vi "4 PulseMeasurements.vi"(2 "4 Pulse Meas Chs":T1={"DI0"="Connector0/DIO0", "DI1"="Connector0/DIO1", "DI2"="Connector0/DIO2", "DI3"="Connector0/DIO3"}, 4 "PulseMeas Timeouts":u32[](array[numeric])=[0, 0, 0, 0]) -> (7 "PulseMeas Packets":u64[](array[numeric]))   [LabVIEW 2010]
uses:
  <vilib>/eio/EIONode/EIONode.xnode
  <vilib>/rvi/eio/nirviEIOImplementation/nirviEIOImplementation.xnode
  <vilib>/rvi/eio/common/nirviEmuClasses.ctl
  <vilib>/rvi/eio/common/nirviEmuTemplateMethod_noerrors.vi
  <vilib>/NI Veristand/FPGA/NI_VS FPGA Support.lvlib
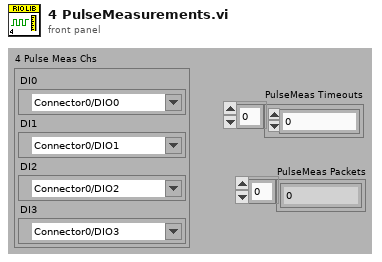
[diagram p1: front panel]
types:
  T1 = cluster{"DI0":refnum<k21>, "DI1":refnum<k21>, "DI2":refnum<k21>, "DI3":refnum<k21>}
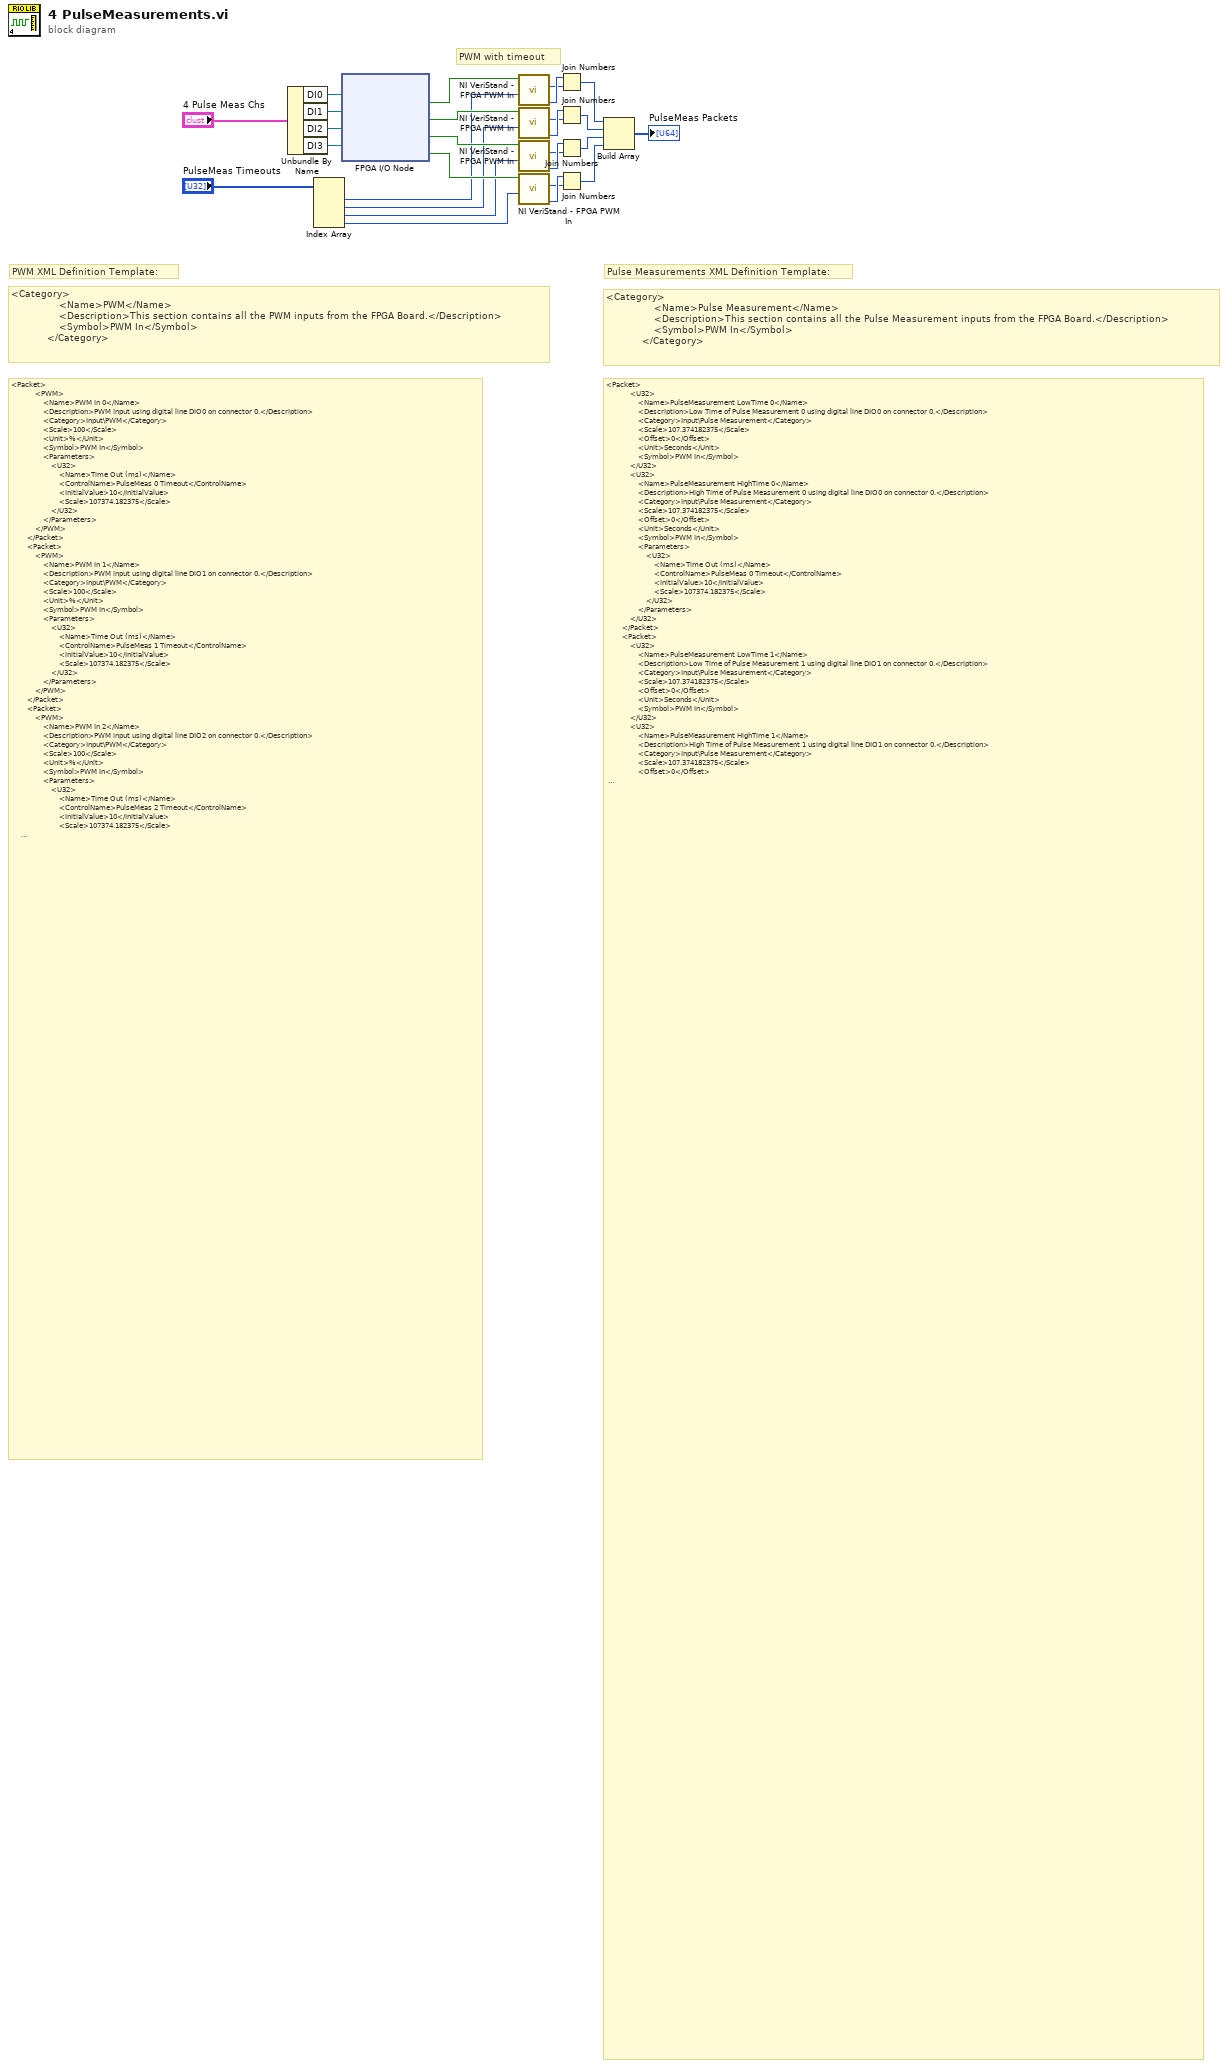
[diagram p0: block diagram]
diagram:
  # "<Category>\n                <Name>PWM</Name>\n                <Description>This section contains all the PWM inputs from the FPGA Board.</Description>\n                <Symbol>PWM In</Symbol>\n            </Category>"
  # "<Category>\n                <Name>Pulse Measurement</Name>\n                <Description>This section contains all the Pulse Measurement inputs from the FPGA Board.</Description>\n                <Symbol>PWM In</Symbol>\n            </Category>"
  # "Pulse Measurements XML Definition Template:"
  # "PWM XML Definition Template:"
  # "<Packet>\n            <PWM>\n                <Name>PWM In 0</Name>\n                <Description>PWM input using digital line DIO0 on connector 0.</Description>\n                <Category>Input\\PWM</Category>\n                <Scale>100</Scale>\n                <Unit>%</Unit>\n                <Symbol>PWM In</Symbol>\n                <Parameters>\n                    <U32>\n                        <Name>Time Out (ms)</Name>\n                        <ControlName>PulseMeas 0 Timeout</ControlName>\n                        <InitialValue>10</InitialValue>\n                        <Scale>107374.182375</Scale>\n                    </U32>\n                </Parameters>\n            </PWM>\n        </Packet>\n        <Packet>\n            <PWM>\n                <Name>PWM In 1</Name>\n                <Description>PWM input using digital line DIO1 on connector 0.</Description>\n                <Category>Input\\PWM</Category>\n                <Scale>100</Scale>\n                <Unit>%</Unit>\n                <Symbol>PWM In</Symbol>\n                <Parameters>\n                    <U32>\n                        <Name>Time Out (ms)</Name>\n                        <ControlName>PulseMeas 1 Timeout</ControlName>\n                        <InitialValue>10</InitialValue>\n                        <Scale>107374.182375</Scale>\n                    </U32>\n                </Parameters>\n            </PWM>\n        </Packet>\n        <Packet>\n            <PWM>\n                <Name>PWM In 2</Name>\n                <Description>PWM input using digital line DIO2 on connector 0.</Description>\n                <Category>Input\\PWM</Category>\n                <Scale>100</Scale>\n                <Unit>%</Unit>\n                <Symbol>PWM In</Symbol>\n                <Parameters>\n                    <U32>\n                        <Name>Time Out (ms)</Name>\n                        <ControlName>PulseMeas 2 Timeout</ControlName>\n                        <InitialValue>10</InitialValue>\n                        <Scale>107374.182375</Scale>\n                    </U32>\n                </Parameters>\n            </PWM>\n        </Packet>\n        <Packet>\n            <PWM>\n                <Name>PWM In 3</Name>\n                <Description>PWM input using digital line DIO3 on connector 0.</Description>\n                <Category>Input\\PWM</Category>\n                <Scale>100</Scale>\n                <Unit>%</Unit>\n                <Symbol>PWM In</Symbol>\n                <Parameters>\n                    <U32>\n                        <Name>Time Out (ms)</Name>\n                        <ControlName>PulseMeas 3 Timeout</ControlName>\n                        <InitialValue>10</InitialValue>\n                        <Scale>107374.182375</Scale>\n                    </U32>\n                </Parameters>\n            </PWM>\n        </Packet>"
  # "<Packet>\n            <U32>\n                <Name>PulseMeasurement LowTime 0</Name>\n                <Description>Low Time of Pulse Measurement 0 using digital line DIO0 on connector 0.</Description>\n                <Category>Input\\Pulse Measurement</Category>\n                <Scale>107.374182375</Scale>\n                <Offset>0</Offset>\n                <Unit>Seconds</Unit>\n                <Symbol>PWM In</Symbol>\n            </U32>\n            <U32>\n                <Name>PulseMeasurement HighTime 0</Name>\n                <Description>High Time of Pulse Measurement 0 using digital line DIO0 on connector 0.</Description>\n                <Category>Input\\Pulse Measurement</Category>\n                <Scale>107.374182375</Scale>\n                <Offset>0</Offset>\n                <Unit>Seconds</Unit>\n                <Symbol>PWM In</Symbol>\n                <Parameters>\n                    <U32>\n                        <Name>Time Out (ms)</Name>\n                        <ControlName>PulseMeas 0 Timeout</ControlName>\n                        <InitialValue>10</InitialValue>\n                        <Scale>107374.182375</Scale>\n                    </U32>\n                </Parameters>\n            </U32>\n        </Packet>\n        <Packet>\n            <U32>\n                <Name>PulseMeasurement LowTime 1</Name>\n                <Description>Low Time of Pulse Measurement 1 using digital line DIO1 on connector 0.</Description>\n                <Category>Input\\Pulse Measurement</Category>\n                <Scale>107.374182375</Scale>\n                <Offset>0</Offset>\n                <Unit>Seconds</Unit>\n                <Symbol>PWM In</Symbol>\n            </U32>\n            <U32>\n                <Name>PulseMeasurement HighTime 1</Name>\n                <Description>High Time of Pulse Measurement 1 using digital line DIO1 on connector 0.</Description>\n                <Category>Input\\Pulse Measurement</Category>\n                <Scale>107.374182375</Scale>\n                <Offset>0</Offset>\n                <Unit>Seconds</Unit>\n                <Symbol>PWM In</Symbol>\n                <Parameters>\n                    <U32>\n                        <Name>Time Out (ms)</Name>\n                        <ControlName>PulseMeas 1 Timeout</ControlName>\n                        <InitialValue>10</InitialValue>\n                        <Scale>107374.182375</Scale>\n                    </U32>\n                </Parameters>\n            </U32>\n        </Packet>\n        <Packet>\n            <U32>\n                <Name>PulseMeasurement LowTime 2</Name>\n                <Description>Low Time of Pulse Measurement 2 using digital line DIO2 on connector 0.</Description>\n                <Category>Input\\Pulse Measurement</Category>\n                <Scale>107.374182375</Scale>\n                <Offset>0</Offset>\n                <Unit>Seconds</Unit>\n                <Symbol>PWM In</Symbol>\n            </U32>\n            <U32>\n                <Name>PulseMeasurement HighTime 2</Name>\n                <Description>High Time of Pulse Measurement 2 using digital line DIO2 on connector 0.</Description>\n                <Category>Input\\Pulse Measurement</Category>\n                <Scale>107.374182375</Scale>\n                <Offset>0</Offset>\n                <Unit>Seconds</Unit>\n                <Symbol>PWM In</Symbol>\n                <Parameters>\n                    <U32>\n                        <Name>Time Out (ms)</Name>\n                        <ControlName>PulseMeas 2 Timeout</ControlName>\n                        <InitialValue>10</InitialValue>\n                        <Scale>107374.182375</Scale>\n                    </U32>\n                </Parameters>\n            </U32>\n        </Packet>\n        <Packet>\n            <U32>\n                <Name>PulseMeasurement LowTime 3</Name>\n                <Description>Low Time of Pulse Measurement 3 using digital line DIO3 on connector 0.</Description>\n                <Category>Input\\Pulse Measurement</Category>\n                <Scale>107.374182375</Scale>\n                <Offset>0</Offset>\n                <Unit>Seconds</Unit>\n                <Symbol>PWM In</Symbol>\n            </U32>\n            <U32>\n                <Name>PulseMeasurement HighTime 3</Name>\n                <Description>High Time of Pulse Measurement 3 using digital line DIO3 on connector 0.</Description>\n                <Category>Input\\Pulse Measurement</Category>\n                <Scale>107.374182375</Scale>\n                <Offset>0</Offset>\n                <Unit>Seconds</Unit>\n                <Symbol>PWM In</Symbol>\n                <Parameters>\n                    <U32>\n                        <Name>Time Out (ms)</Name>\n                        <ControlName>PulseMeas 3 Timeout</ControlName>\n                        <InitialValue>10</InitialValue>\n                        <Scale>107374.182375</Scale>\n                    </U32>\n                </Parameters>\n            </U32>\n        </Packet>"
  # "PWM with timeout"
  n1 = Unbundle By Name("4 Pulse Meas Chs") -> ("DI0"=w1:refnum<k21>, "DI1"=w2:refnum<k21>, "DI2"=w3:refnum<k21>, "DI3"=w4:refnum<k21>)
  n2 = Index Array(array="PulseMeas Timeouts") -> (element #1=w6:u32, element #2=w7:u32, element #3=w8:u32, element #4=w9:u32)  [unwired: 4 in]
  n3 = xnode "FPGA I/O Node"("FPGA I/O In"=w1, "FPGA I/O In"=w2, "FPGA I/O In"=w3, "FPGA I/O In"=w4) -> ("I/O Item"=w11:bool, "I/O Item"=w14:bool, "I/O Item"=w15:bool, "I/O Item"=w16:bool)  [unwired: 4 out]
  n4 = call <vilib>:"NI VeriStand - FPGA PWM In.vi"("Time Out"=w6, "Value"=w11) -> ("High time"=w13:u32, "Low Time"=w12:u32)  [unwired: 8 out]
  n5 = call <vilib>:"NI VeriStand - FPGA PWM In.vi"("Time Out"=w7, "Value"=w14) -> ("High time"=w22:u32, "Low Time"=w17:u32)  [unwired: 8 out]
  n6 = call <vilib>:"NI VeriStand - FPGA PWM In.vi"("Time Out"=w8, "Value"=w15) -> ("High time"=w21:u32, "Low Time"=w18:u32)  [unwired: 8 out]
  n7 = call <vilib>:"NI VeriStand - FPGA PWM In.vi"("Time Out"=w9, "Value"=w16) -> ("High time"=w20:u32, "Low Time"=w19:u32)  [unwired: 8 out]
  n8 = Join Numbers(hi=w13, lo=w12) -> ((hi.lo)=w23:u64)
  n9 = Join Numbers(hi=w22, lo=w17) -> ((hi.lo)=w24:u64)
  n10 = Join Numbers(hi=w21, lo=w18) -> ((hi.lo)=w25:u64)
  n11 = Join Numbers(hi=w20, lo=w19) -> ((hi.lo)=w26:u64)
  n12 = Build Array(w23, w24, w25, w26) -> (→"PulseMeas Packets":u64[])
